vi "LWXPS_Close.vi"(3 "LabVIEW error IN":errorcluster caption="error in", 5 "XPS Reference":refnum<k24>) -> (0 "LabVIEW error OUT":errorcluster caption="error out", 1 "Returned Error code":i32)   [LabVIEW 2020]
uses:
  C:/Users/loasis.BELLANET/Downloads/XPS-UNIFIED/LabVIEW VIs/LabVIEW Source Code/Dll/Newport.XPS.CommandInterface.dll
  Users/loasis.BELLANET/Downloads/XPS-UNIFIED/LabVIEW VIs/LabVIEW Source Code/Dll/Newport.XPS.CommandInterface.dll
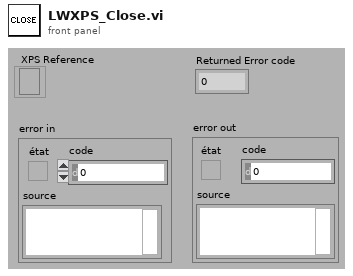
[diagram p1: front panel]
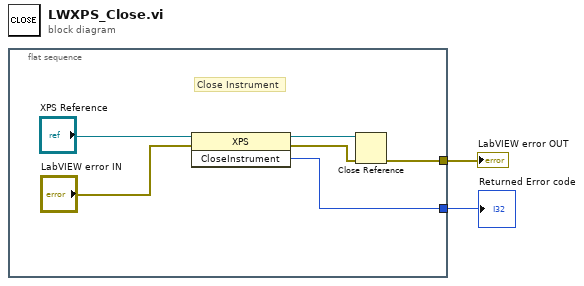
[diagram p0: block diagram]
diagram:
  n1 = flat-sequence {
    tunnel: [w4] -> w2
    tunnel: [w3] -> w1
    frame #0 {
      # "Close Instrument"
      n2 = invoke class="XPS" method="CloseInstrument"(reference="XPS Reference", error in="LabVIEW error IN") -> (reference out=w5:refnum<k24>, error out=w6:errorcluster, "CloseInstrument"=w3:i32)  [unwired: 1 in]
      n3 = Close Reference(reference=w5, error in (no error)=w6) -> (error out=w4:errorcluster)
    }
  }
  "LabVIEW error OUT" <- w2
  "Returned Error code" <- w1
